vi "Calibration Complete.vi"(8 "error in":errorcluster, 11 "Pcal GUI in":refnum<class "Pcal GUI.lvclass">) -> (0 "error out":errorcluster, 3 "Pcal GUI out":refnum<class "Pcal GUI.lvclass">)   [LabVIEW 2015, in "Pcal GUI.lvclass"]
uses:
  Pcal GUI.lvclass
  Pcal GUI.lvclass/Pcal GUI.ctl
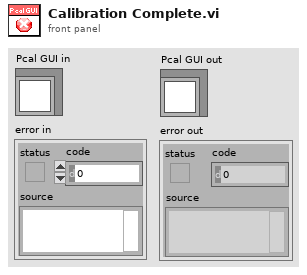
[diagram p1: front panel]
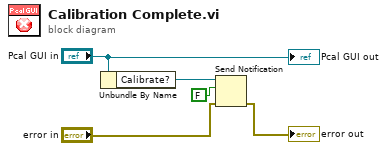
[diagram p0: block diagram]
diagram:
  n1 = Unbundle By Name("Pcal GUI in") -> ("Calibrate?"=w4:refnum<notifier>)
  n2 = Send Notification(notification=FALSE, notifier=w4, error in (no error)="error in") -> (error out=→"error out":errorcluster)  [unwired: 1 out]
  "Pcal GUI out" <- "Pcal GUI in"
